vi "Ex4.vi"() -> ()   [LabVIEW 2010]
uses:
  <userlib>/ROSforLV_0.1/ROS/Code/JointPositions.ctl
  <userlib>/ROSforLV_0.1/ROS/Code/Slider.ctl
panel:
  in  "Loop Rate (Hz)":dbl
  in  "Joint Positions":T1 {"left_w2" scale=-180.0..180.0; "left_w1" scale=-180.0..180.0; "left_w0" scale=-180.0..180.0; "left_e1" scale=-180.0..180.0; "left_e0" scale=-180.0..180.0; "left_s1" scale=-180.0..180.0; "left_s0" scale=-180.0..180.0; "right_s1" scale=-180.0..180.0; "right_s0" scale=-180.0..180.0; "right_w2" scale=-180.0..180.0; "right_e1" scale=-180.0..180.0; "right_e0" scale=-180.0..180.0; "right_w0" scale=-180.0..180.0; "right_w1" scale=-180.0..180.0}
  in  "stop":bool
  # "Control Baxter's Arms using the supplied Position Controller"
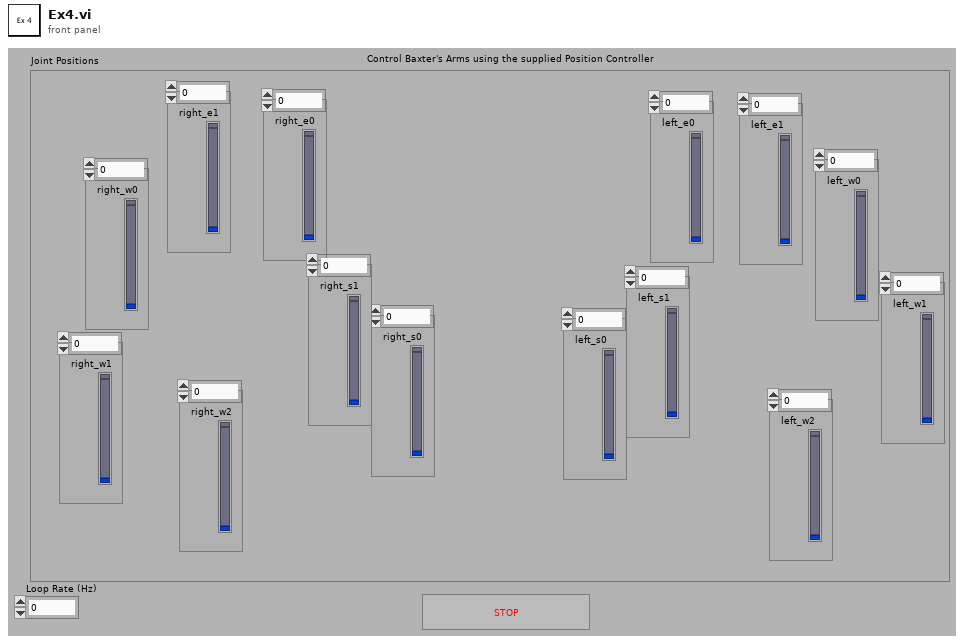
[diagram p1: front panel]
types:
  T1 = typedef "JointPositions.ctl" = cluster{"left_e0":T2, "left_e1":T2, "left_s0":T2, "left_s1":T2, "left_w0":T2, "left_w1":T2, "left_w2":T2, "right_e0":T2, "right_e1":T2, "right_s0":T2, "right_s1":T2, "right_w0":T2, "right_w1":T2, "right_w2":T2}
  T2 = typedef "Slider.ctl" = dbl
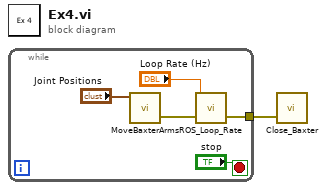
[diagram p0: block diagram]
diagram:
  n1 = while {
    tunnel: [w3] -> w1
    stop <- "stop" stop-if-true
    n2 = call <userlib>:"MoveBaxterArms.vi"("Parameters"="Joint Positions") -> ("error out"=w4:errorcluster)  [unwired: 5 in]
    n3 = call <userlib>:"ROS_Loop_Rate.vi"("Loop Rate (Hz)"="Loop Rate (Hz)", "error in"=w4) -> ("error out"=w3:errorcluster)  [unwired: 3 in, 1 out]
  }
  n4 = call <userlib>:"Close_Baxter.vi"("error in"=w1) -> ()  [unwired: 3 in, 1 out]
